vi "Configure Voltage Limit Level.vi"(8 "error in":errorcluster, 9 "Level(V)":dbl min=0.0 max=610.0, 10 "Slew Type":u16(ring) caption="Type" items=["High", "Low"], 11 "VISA resource name":refnum<visa-resource-name>) -> (0 "error out":errorcluster, 3 "VISA resource name out":refnum<visa-resource-name>)   [LabVIEW 2018, in "IT-M3100.lvlib"]
doc: "This command sets the maximum setting voltage limit and the minimum setting voltage limit of the power supply.\n<b>Type</b>\n0:High\n1:Low\n<b>Level(V)</b>\n0-610"
uses:
  IT-M3100.lvlib
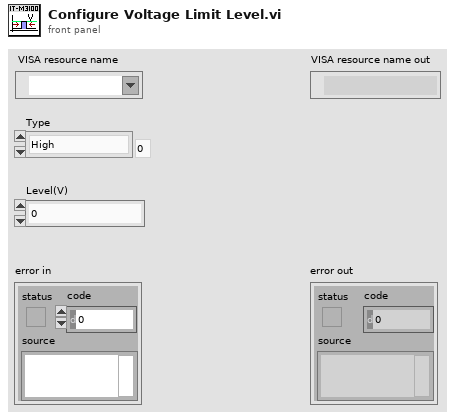
[diagram p1: front panel]
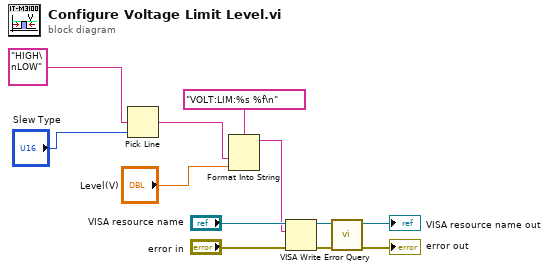
[diagram p0: block diagram]
diagram:
  n1 = Pick Line(multi-line string="HIGH\nLOW", line index="Slew Type") -> (output string=w1:string)  [unwired: 1 in]
  n2 = Format Into String(format string="VOLT:LIM:%s %f\n", w1, "Level(V)") -> (resulting string=w5:string)  [unwired: 2 in, 1 out]
  n3 = VISA Write(VISA resource name="VISA resource name", write buffer=w5, error in (no error)="error in") -> (VISA resource name out=w9:refnum<visa-resource-name>, error out=w10:errorcluster)  [unwired: 1 out]
  n4 = call "Error Query.vi"("error in"=w10, "VISA resource name"=w9) -> ("error out"=→"error out":errorcluster, "VISA resource name out"=→"VISA resource name out":refnum<visa-resource-name>)  [unwired: 6 in, 2 out]
